vi "Calculate Time Left.vi"(8 "Interval":dbl=30.0 caption="PROFILER (SEC)", 10 "Total Samples":i32=10, 11 "Acquired Samples":i32) -> (0 "MINS Left":dbl format="%_3g", 3 "HRS Left":dbl)   [LabVIEW 2017]
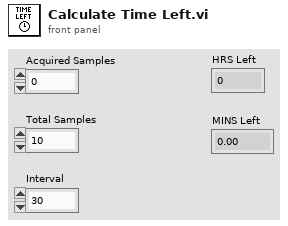
[diagram p1: front panel]
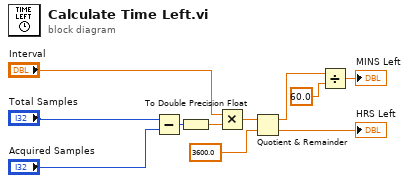
[diagram p0: block diagram]
diagram:
  n1 = Subtract(x="Total Samples", y="Acquired Samples") -> (x-y=w11:i32)
  n2 = To Double Precision Float(number=w11) -> (double precision float=w10:dbl)
  n3 = Multiply(x="Interval", y=w10) -> (x*y=w9:dbl)
  n4 = Quotient & Remainder(x=w9, y=3600.0) -> (x-y*floor(x/y)=w6:dbl, floor(x/y)=→"HRS Left":dbl)
  n5 = Divide(x=w6, y=60.0) -> (x/y=→"MINS Left":dbl)
